vi "Decimate XY Absolute.vi"(6 "Width":i32, 8 "error in (no error)":errorcluster, 9 "Xmin":i32, 10 "Xmax":i32, 11 "Data to Decimate":cluster{"X":dbl[], "Y":dbl[]}[](array[cluster])) -> (0 "error out":errorcluster, 3 "Decimated Data":cluster{"X":dbl[], "Y":dbl[]}[](array[cluster]))   [LabVIEW 2022 SP3, in "Decimation.lvlib"]
doc: "Decimate XY array to optimize the density of points per pixel to 2 : Min & Max per pixel."
uses:
  Decimation.lvlib
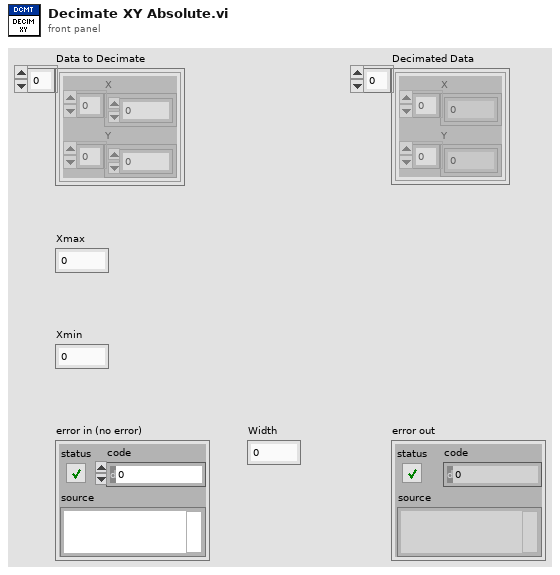
[diagram p1: front panel]
types:
  T1 = cluster{"Decimated Data":dbl[], "Decimated Data":dbl[]}
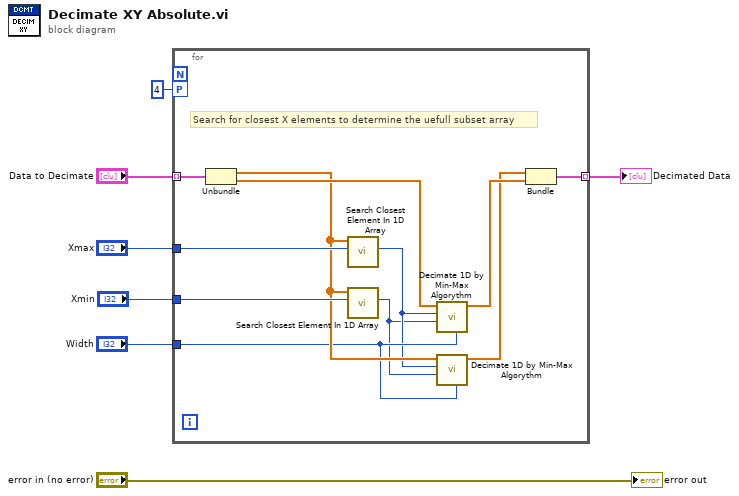
[diagram p0: block diagram]
diagram:
  n1 = for {
    tunnel: "Data to Decimate" -> [w18] mode=indexing
    tunnel: "Xmin" -> [w17]
    tunnel: "Xmax" -> [w16]
    tunnel: [w15] -> w3 mode=indexing
    workers-P: 4 -> [_]
    tunnel: "Width" -> [w10]
    # "Search for closest X elements to determine the uefull subset array"
    n2 = Unbundle(w18) -> ("X"=w12:dbl[], "Y"=w14:dbl[])
    n3 = call "Search Closest Element In 1D Array.vi"("Desired element"=w16, "1D Array"=w12) -> ("Closest Index"=w9:i32)  [unwired: 8 in, 1 out]
    n4 = call "Search Closest Element In 1D Array.vi"("Desired element"=w17, "1D Array"=w12) -> ("Closest Index"=w8:i32)  [unwired: 8 in, 1 out]
    n5 = call "Decimate 1D by Min-Max Algorythm.vi"("Width"=w10, "Min Index"=w8, "Max Index"=w9, "Data To Decimate"=w14) -> ("Decimated Data"=w13:dbl[])  [unwired: 6 in, 1 out]
    n6 = call "Decimate 1D by Min-Max Algorythm.vi"("Width"=w10, "Min Index"=w8, "Max Index"=w9, "Data To Decimate"=w12) -> ("Decimated Data"=w11:dbl[])  [unwired: 6 in, 1 out]
    n7 = Bundle("Decimated Data"=w11, "Decimated Data"=w13) -> (w15:T1)  [unwired: 1 in]
  }
  "Decimated Data" <- w3
  "error out" <- "error in (no error)"
